vi "setBufferSize.vi"(8 "error in (no error)":errorcluster, 10 "bufferSize":u32=50000, 11 "Electrometer in":refnum<class "Electrometer.lvclass">) -> (0 "error out":errorcluster, 3 "Electrometer out":refnum<class "Electrometer.lvclass">)   [LabVIEW 2016, in "Electrometer.lvclass"]
uses:
  Electrometer.lvclass
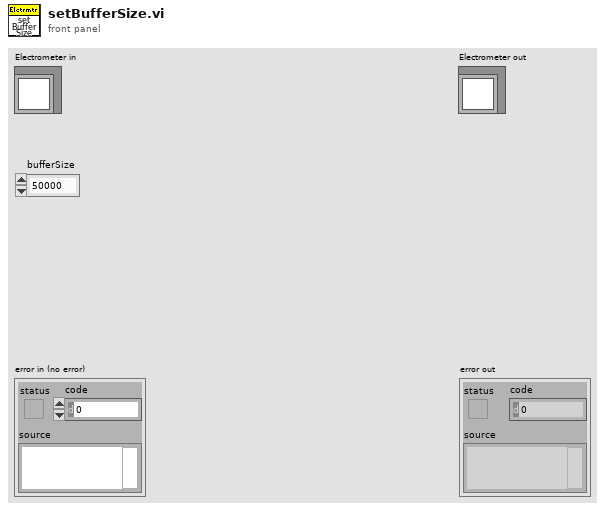
[diagram p1: front panel]
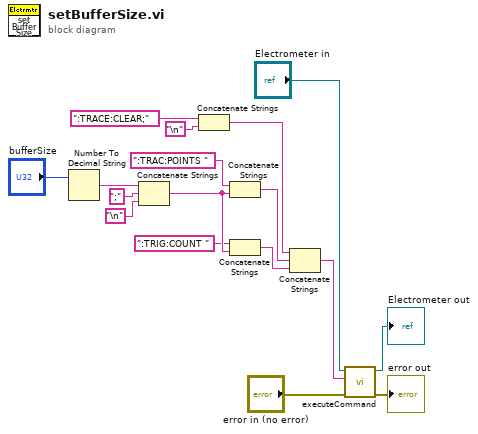
[diagram p0: block diagram]
diagram:
  n1 = Number To Decimal String(number="bufferSize") -> (decimal integer string=w11:string)  [unwired: 1 in]
  n2 = Concatenate Strings(w11, ";" ("string"), "\n") -> (w9:string)
  n3 = Concatenate Strings(":TRACE:CLEAR;" ("command"), "\n") -> (w2:string)
  n4 = Concatenate Strings(":TRAC:POINTS " ("command"), w9) -> (w8:string)
  n5 = Concatenate Strings(":TRIG:COUNT " ("command"), w9) -> (w7:string)
  n6 = Concatenate Strings(w2, w8, w7) -> (w6:string)
  n7 = call "executeCommand.vi"("error in (no error)"="error in (no error)", "command"=w6, "Electrometer in"="Electrometer in") -> ("error out"=→"error out":errorcluster, "Electrometer out"=→"Electrometer out":refnum<class "Electrometer.lvclass">)  [unwired: 7 in]
